vi "execute.vi"(8 "error in (no error)":errorcluster, 9 "trajectory in":refnum<class "GenericComponent.lvclass">, 10 "imaging mode in":refnum<class "GenericComponent.lvclass">, 11 "AdapterMH100804ImagingModeToTrajectory in":refnum<class "AdapterMH100804ImagingModeToTrajectory.lvclass">) -> (0 "error out":errorcluster, 1 "B out":refnum<class "GenericComponent.lvclass">, 2 "A out":refnum<class "GenericComponent.lvclass">, 3 "AdapterMH100804ImagingModeToTrajectory out":refnum<class "AdapterMH100804ImagingModeToTrajectory.lvclass">)   [LabVIEW 2010, in "AdapterMH100804ImagingModeToTrajectory.lvclass"]
uses:
  AdapterMH100804ImagingModeToTrajectory.lvclass
  common/classes/GenericComponent/GenericComponent/GenericComponent.lvclass
  Trajectory/TrajectoryMG100122AODFrameScan/TrajectoryMG100122AODFrameScan/TrajectoryMG100122AODFrameScan.lvclass
  ImagingMode/ImagingModeDL090130Frame/ImagingModeDL090130Frame/ImagingModeDL090130Frame.lvclass
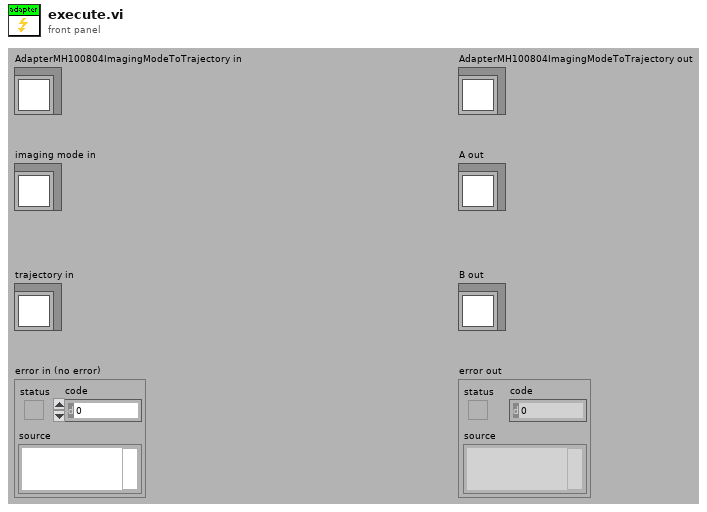
[diagram p1: front panel]
types:
  T1 = enum16{"frame rate", "line-scan time", "pixel-dwell time"}
  T2 = typedef "ImagingModeDL090130Frame.lvclass/speed_parameter_cluster.ctl" = enum16{"frame rate", "line-scan time", "pixel-dwell time"}
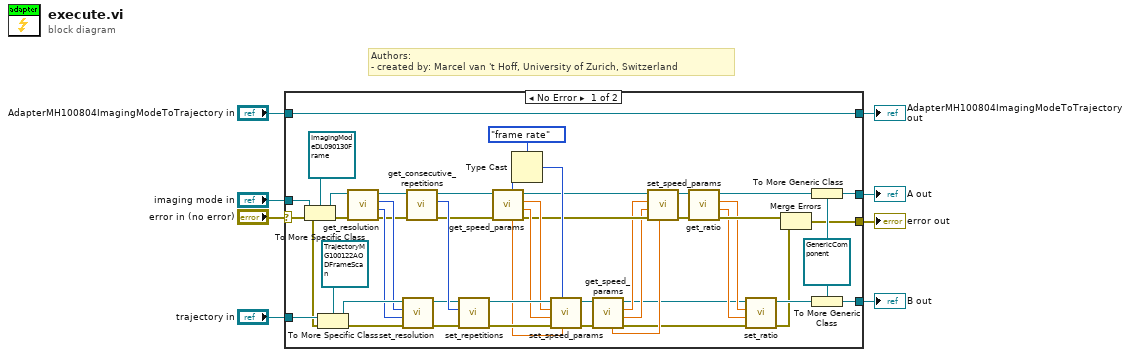
[diagram p0: block diagram]
diagram:
  # "Authors: \n- created by: Marcel van 't Hoff, University of Zurich, Switzerland"
  n1 = case shown="No Error" "error in (no error)" {
    selector: "error in (no error)" -> [w41 w58]
    tunnel: "imaging mode in" -> [w53 w59]
    tunnel: "AdapterMH100804ImagingModeToTrajectory in" -> [w56 w60]
    tunnel: [w56 w60] -> w5
    tunnel: [w44 w59] -> w4
    tunnel: [w30 w58] -> w3
    tunnel: [w51 w57] -> w2
    tunnel: "trajectory in" -> [w50 w57]
    frame No Error {
      w43 = refnum<class "GenericComponent.lvclass"> refnum ("GenericComponent.lvclass")
      n2 = To More Specific Class(target class=refnum<class "ImagingModeDL090130Frame.lvclass"> refnum ("ImagingModeDL090130Frame.lvclass"), reference=w53, error in=w41) -> (specific class reference=w52:refnum<class "ImagingModeDL090130Frame.lvclass">, error out=w54:errorcluster)
      n3 = To More Specific Class(target class=refnum<class "TrajectoryMG100122AODFrameScan.lvclass"> refnum ("TrajectoryMG100122AODFrameScan.lvclass"), reference=w50, error in=w41) -> (specific class reference=w47:refnum<class "TrajectoryMG100122AODFrameScan.lvclass">, error out=w48:errorcluster)
      n4 = call-dynamic "get_resolution.vi"("error in (no error)"=w54, "ImagingModeDL090130Frame in"=w52) -> ("error out"=w38:errorcluster, "y resolution"=w46:i32, "x resolution"=w42:i32, "ImagingModeDL090130Frame out"=w37:refnum<class "ImagingModeDL090130Frame.lvclass">)  [unwired: 6 in]
      n5 = call-dynamic "set_resolution.vi"("error in (no error)"=w48, "y resolution"=w46, "x resolution"=w42, "TrajectoryMG100122AODFrameScan in"=w47) -> ("error out"=w40:errorcluster, "TrajectoryMG100122AODFrameScan out"=w39:refnum<class "TrajectoryMG100122AODFrameScan.lvclass">)  [unwired: 6 in]
      n6 = call-dynamic "get_consecutive_repetitions.vi"("error in (no error)"=w38, "ImagingModeDL090130Frame in"=w37) -> ("error out"=w34:errorcluster, "number of consecutive repetitions"=w45:i32, "ImagingModeDL090130Frame out"=w35:refnum<class "ImagingModeDL090130Frame.lvclass">)  [unwired: 7 in]
      n7 = call-dynamic "set_repetitions.vi"("error in (no error)"=w40, "repetitions"=w45, "GenericTrajectory in"=w39) -> ("error out"=w28:errorcluster, "GenericTrajectory out"=w29:refnum<class "TrajectoryMG100122AODFrameScan.lvclass">)  [unwired: 7 in]
      n8 = call-dynamic "get_speed_params.vi"("error in (no error)"=w34, "ImagingModeDL090130Frame in"=w35) -> ("error out"=w21:errorcluster, "line-scan time"=w26:dbl[unit], "frame rate"=w27:dbl[unit], "ImagingModeDL090130Frame out"=w23:refnum<class "ImagingModeDL090130Frame.lvclass">, "pixel dwell time"=w25:dbl[unit], "which one is correct for sure?"=w33:T2)  [unwired: 4 in]
      n9 = Type Cast(type=T1."frame rate" ("speed param"), x=w33) -> (*(type *) &x=w24:T1)
      n10 = call-dynamic "set_speed_params.vi"("pixel-dwell time"=w25, "speed param"=w24, "error in (no error)"=w28, "line-scan time"=w26, "frame rate"=w27, "TrajectoryMG100122AODFrameScan in"=w29) -> ("error out"=w18:errorcluster, "TrajectoryMG100122AODFrameScan out"=w19:refnum<class "TrajectoryMG100122AODFrameScan.lvclass">)  [unwired: 4 in]
      n11 = call-dynamic "get_speed_params.vi"("error in (no error)"=w18, "TrajectoryMG100122AODFrameScan in"=w19) -> ("error out"=w10:errorcluster, "line-scan time"=w16:dbl[unit], "frame rate"=w17:dbl[unit], "TrajectoryMG100122AODFrameScan out"=w12:refnum<class "TrajectoryMG100122AODFrameScan.lvclass">, "pixel-dwell time"=w15:dbl[unit])  [unwired: 5 in]
      n12 = call-dynamic "set_speed_params.vi"("pixel-dwell time"=w15, "error in (no error)"=w21, "line-scan time"=w16, "frame rate"=w17, "ImagingModeDL090130Frame in"=w23) -> ("error out"=w20:errorcluster, "ImagingModeDL090130Frame out"=w22:refnum<class "ImagingModeDL090130Frame.lvclass">)  [unwired: 5 in]
      n13 = call-dynamic "get_ratio.vi"("error in (no error)"=w20, "ImagingModeDL090130Frame in"=w22) -> ("error out"=w31:errorcluster, "y ratio factor"=w13:dbl, "x ratio factor"=w14:dbl, "ImagingModeDL090130Frame out"=w36:refnum<class "ImagingModeDL090130Frame.lvclass">)  [unwired: 6 in]
      n14 = call-dynamic "set_ratio.vi"("error in (no error)"=w10, "y"=w13, "x"=w14, "TrajectoryMG100122AODFrameScan in"=w12) -> ("error out"=w9:errorcluster, "TrajectoryMG100122AODFrameScan out"=w11:refnum<class "TrajectoryMG100122AODFrameScan.lvclass">)  [unwired: 6 in]
      n15 = Merge Errors(w31, w9) -> (w30:errorcluster)
      n16 = To More Generic Class(target class=w43, reference=w36) -> (generic class reference=w44:refnum<class "GenericComponent.lvclass">)
      n17 = To More Generic Class(target class=w43, reference=w11) -> (generic class reference=w51:refnum<class "GenericComponent.lvclass">)
    }
    frame Error {
    }
  }
  "error out" <- w3
  "AdapterMH100804ImagingModeToTrajectory out" <- w5
  "A out" <- w4
  "B out" <- w2
